vi "FGVHdtServer.vi"(6 "NewData":T1={"OwnerVi"="", "hdt.int.s.transferSource"=2, "Used"=TRUE} {"hdt.int.s.transferSource" items=["memoryChan1", "memoryChan2", "processVarFixedNoPts", "processVarStream", "systemID"]}, 7 "Enum":T2, 8 "error in":errorcluster, 9 "UsedIn":bool[](array[boolean]), 10 "HDTTransferSourceIn":u8[](array[ring]) items=["memoryChan1", "memoryChan2", "processVarFixedNoPts", "processVarStream", "systemID"], 11 "OwnerViIn":string[](array[string])) -> (0 "error out":errorcluster, 1 "UsedOut":bool[](array[boolean]), 2 "HdtTransferSourceOut":u8[](array[ring]) items=["memoryChan1", "memoryChan2", "processVarFixedNoPts", "processVarStream"], 3 "OwnerViOut":string[](array[string]))   [LabVIEW 2016]
uses:
  controls/EnumFGVHDT.ctl
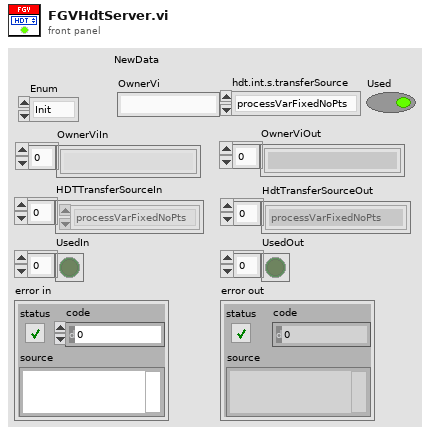
[diagram p1: front panel]
types:
  T1 = cluster{"OwnerVi":string, "hdt.int.s.transferSource":u8, "Used":bool}
  T2 = typedef "EnumFGVHDT.ctl" = enum16{"Init", "Read", "Write", "Push", "Pop"}
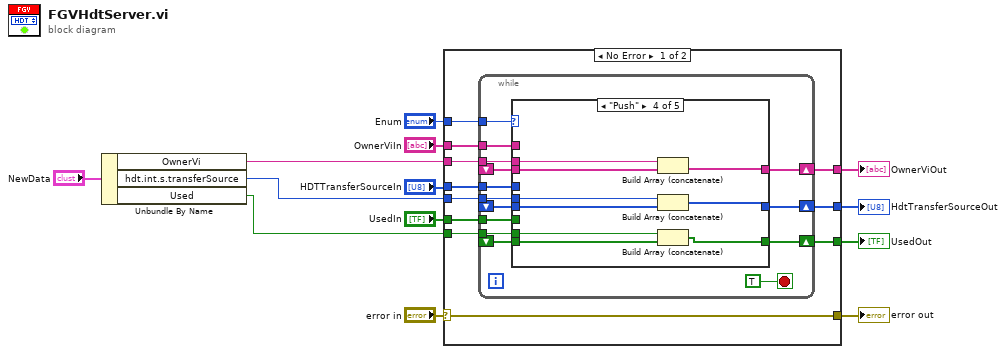
[diagram p0: block diagram]
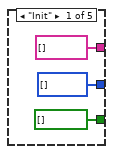
[diagram p2: hidden frame]
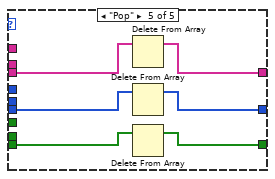
[diagram p5: hidden frame]
diagram:
  n1 = Unbundle By Name("NewData") -> ("OwnerVi"=w3:string, "hdt.int.s.transferSource"=w2:u8, "Used"=w1:bool)
  n2 = case shown="No Error" "error in" {
    selector: "error in" -> [w23 w66]
    tunnel: "Enum" -> [w24 _]
    tunnel: [w23 w66] -> w13
    tunnel: "HDTTransferSourceIn" -> [w21 w64]
    tunnel: [w22 w64] -> w10
    tunnel: "UsedIn" -> [w20 w65]
    tunnel: [w19 w65] -> w8
    tunnel: "OwnerViIn" -> [w17 w63]
    tunnel: [w18 w63] -> w6
    tunnel: w3 -> [w16 _]
    tunnel: w2 -> [w15 _]
    tunnel: w1 -> [w14 _]
    frame No Error {
      n3 = while {
        tunnel: w24 -> [w37]
        shift-right: [w36] -> w22
        shift-left: _ -> [w34]
        tunnel: w21 -> [w35]
        tunnel: w20 -> [w33]
        shift-right: [w32] -> w19
        shift-left: _ -> [w31]
        tunnel: w17 -> [w29]
        shift-right: [w30] -> w18
        shift-left: _ -> [w28]
        tunnel: w16 -> [w27]
        tunnel: w15 -> [w26]
        tunnel: w14 -> [w25]
        stop <- TRUE stop-if-true
        n4 = case shown="\"Push\"" w37 {
          tunnel: [u8[] [] ("ArrayIn") w44 w47 w54 w60] -> w36
          tunnel: w35 -> [_ _ w47 _ _]
          tunnel: w34 -> [_ w44 _ w53 w57]
          tunnel: w33 -> [_ _ w46 _ _]
          tunnel: [bool[] [] ("UsedIn") w43 w46 w51 w59] -> w32
          tunnel: w31 -> [_ w43 _ w52 w58]
          tunnel: [string[] [] ("OwnerViIn") w42 w45 w56 w61] -> w30
          tunnel: w29 -> [_ _ w45 _ _]
          tunnel: w28 -> [_ w42 _ w55 w62]
          tunnel: w27 -> [_ _ _ w50 _]
          tunnel: w26 -> [_ _ _ w49 _]
          tunnel: w25 -> [_ _ _ w48 _]
          frame "Init" {
          }
          frame "Read", Default {
          }
          frame "Write" {
          }
          frame "Push" {
            n5 = Build Array (concatenate)(w50, w55) -> (w56:string[])
            n6 = Build Array (concatenate)(w49, w53) -> (w54:u8[])
            n7 = Build Array (concatenate)(w48, w52) -> (w51:bool[])
          }
          frame "Pop" {
            n8 = Delete From Array(array=w62) -> (array with subset deleted=w61:string[])  [unwired: 2 in, 1 out]
            n9 = Delete From Array(array=w57) -> (array with subset deleted=w60:u8[])  [unwired: 2 in, 1 out]
            n10 = Delete From Array(array=w58) -> (array with subset deleted=w59:bool[])  [unwired: 2 in, 1 out]
          }
        }
      }
    }
    frame Error {
    }
  }
  "error out" <- w13
  "UsedOut" <- w8
  "HdtTransferSourceOut" <- w10
  "OwnerViOut" <- w6
